vi "Dialog - Select Channel Dialog.vi"(8 "error in (no error)":errorcluster, 9 "Allow Section Selection (F)":bool, 10 "Initial Selection":T1[](array[typedef]) format="%.0x", 11 "Root Item Ref":T1 format="%.0x") -> (0 "error out":errorcluster, 1 "Canceled":bool, 3 "Selected Channel Refs":T1[](array[typedef]) format="%.0x")   [LabVIEW 2016, in "UDP-Custom-Device System Explorer.lvlib"]
doc: "Standard Channel Select Dialog that allows the user to select which TimeStamp channel to use for the header information."
uses:
  UDP-Custom-Device System Explorer.lvlib
  <vilib>/NI Veristand/Custom Device API/Custom Device Item Ref.ctl
  <vilib>/NI VeriStand/Custom Device API/Custom Device API.lvlib
  <vilib>/NI VeriStand/Custom Device Tools/Custom Device Utility Library/Custom Device Utility Library.lvlib
panel:
  in  "Channels":string[](tree)
  in  "Cancel":bool
  in  "OK":bool
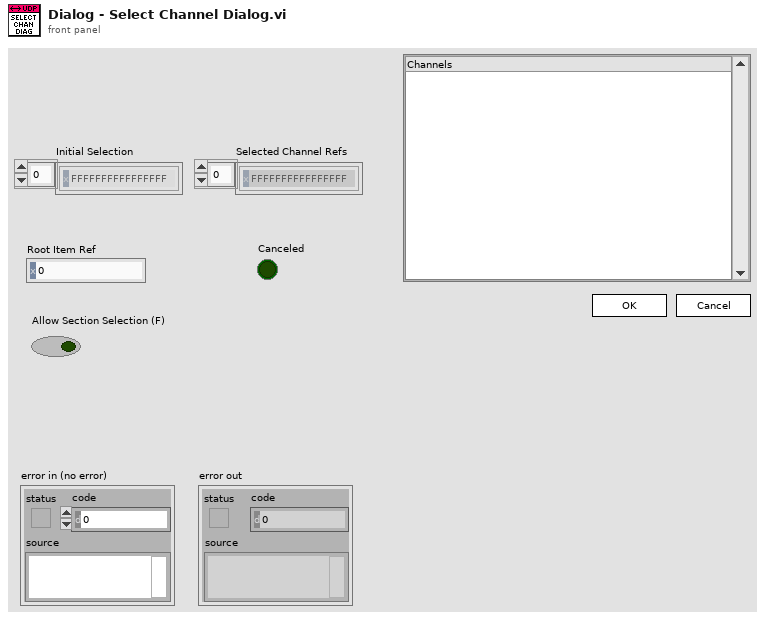
[diagram p1: front panel]
types:
  T1 = typedef "Custom Device API.lvlib/Custom Device Item Ref.ctl" = u64
  T2 = typedef "Custom Device API.lvlib/Custom Device Item Info.ctl" = cluster{"Name":string, "Is Channel":bool, "GUID":string, "Is Waveform":bool}
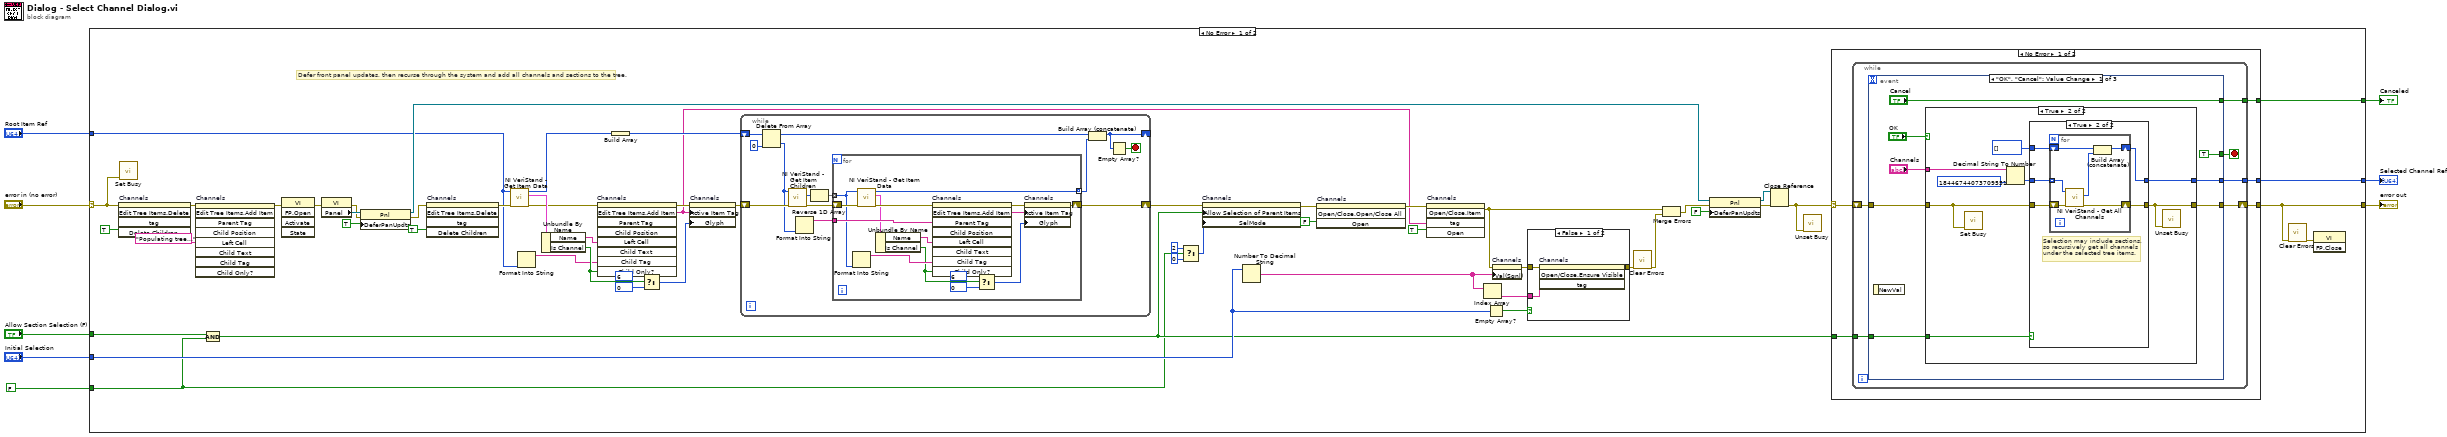
[diagram p0: block diagram]
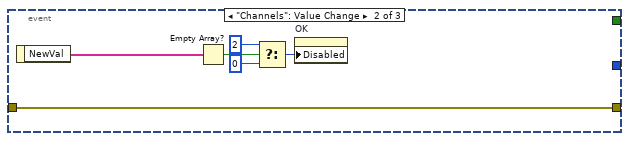
[diagram p5: hidden frame]
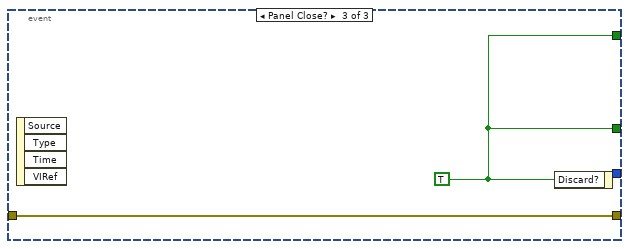
[diagram p6: hidden frame]
diagram:
  n1 = case shown="No Error" "error in (no error)" {
    selector: "error in (no error)" -> [w10 w146]
    tunnel: "Initial Selection" -> [w26 _]
    tunnel: "Allow Section Selection (F)" -> [w16 _]
    tunnel: [w46 w146] -> w5
    tunnel: [w47 _] -> w4
    tunnel: [w44 _] -> w3
    tunnel: "Root Item Ref" -> [w31 _]
    tunnel: FALSE ("Allow Multiple Selection (F)") -> [w11 _]
    frame No Error {
      # "Defer front panel updates, then recurse through the system and add all channels and sections to the tree."
      n2 = invoke on="Channels" class="Tree (strict)" method="Edit Tree Items.Delete"(error in=w10, "Delete Children"=TRUE ("Delete Children?")) -> (error out=w63:errorcluster)  [unwired: 3 in, 4 out]
      n3 = call <vilib>:"Set Busy.vi"("error in (no error)"=w10) -> ()  [unwired: 3 in, 8 out]
      n4 = invoke on="Channels" class="Tree (strict)" method="Edit Tree Items.Add Item"(error in=w63, "Left Cell"="Populating tree..." ("Tag")) -> (error out=w60:errorcluster)  [unwired: 7 in, 8 out]
      n5 = Compound Arithmetic op=AND(w16, w11) -> (w12:bool)
      n6 = invoke class="VI" method="FP.Open"(error in=w60) -> (error out=w58:errorcluster)  [unwired: 4 in, 4 out]
      n7 = property class="VI"(error in=w58) -> (error out=w56:errorcluster, "Panel"=w57:refnum<vi>)  [unwired: 1 in, 1 out]
      n8 = property class="Pnl"(reference=w57, error in=w56, "DeferPanUpdts"=TRUE ("Defer Panel Updates")) -> (reference out=w50:refnum<vi>, error out=w54:errorcluster)
      n9 = invoke on="Channels" class="Tree (strict)" method="Edit Tree Items.Delete"(error in=w54, "Delete Children"=TRUE ("Delete Children?")) -> (error out=w32:errorcluster)  [unwired: 3 in, 4 out]
      n10 = call <vilib>:"NI VeriStand - Get Item Data.vi"("error in (no error)"=w32, "Item Ref in"=w31) -> ("error out"=w35:errorcluster, "Item Info"=w37:T2, "Item Ref out"=w33:T1)  [unwired: 7 out]
      n11 = Format Into String(w31) -> (resulting string=w36:string)  [unwired: 3 in, 1 out]
      n12 = Unbundle By Name(w37) -> ("Name"=w38:string, "Is Channel"=w42:bool)
      n13 = invoke on="Channels" class="Tree (strict)" method="Edit Tree Items.Add Item"(error in=w35, "Left Cell"=w38, "Child Tag"=w36, "Child Only?"=w42) -> (error out=w39:errorcluster, "Edit Tree Items:Add Item"=w17:string)  [unwired: 5 in, 7 out]
      n14 = Build Array(w33) -> (w53:T1[])
      n15 = Select(t=6, s=w42, f=0) -> (s? t:f=w43:i32)
      n16 = property on="Channels" class="Tree (strict)"(error in=w39, "Active Item Tag"=w17, "Glyph"=w43) -> (error out=w34:errorcluster)  [unwired: 1 in, 1 out]
      n17 = while {
        shift-right: [w122] -> w52
        shift-left: w34 -> [w127]
        shift-right: [w126] -> _
        shift-left: w53 -> [w130]
        stop <- w125 stop-if-true
        n18 = Delete From Array(array=w130, index=0) -> (deleted portion=w121:T1, array with subset deleted=w128:T1[])  [unwired: 1 in]
        n19 = call <vilib>:"NI VeriStand - Get Item Children.vi"("error in (no error)"=w127, "Item Ref in"=w121) -> ("error out"=w124:errorcluster, "Child Refs"=w119:T1[])  [unwired: 8 out]
        n20 = Format Into String(w121) -> (resulting string=w120:string)  [unwired: 3 in, 1 out]
        n21 = Reverse 1D Array(array=w119) -> (reversed array=w118:T1[])
        n22 = for {
          shift-right: [w135] -> w122
          shift-left: w124 -> [w144]
          tunnel: w118 -> [w141] mode=indexing
          tunnel: [w142] -> w123 mode=indexing
          tunnel: w120 -> [w145]
          n23 = Format Into String(w141) -> (resulting string=w140:string)  [unwired: 3 in, 1 out]
          n24 = call <vilib>:"NI VeriStand - Get Item Data.vi"("error in (no error)"=w144, "Item Ref in"=w141) -> ("error out"=w143:errorcluster, "Item Info"=w139:T2, "Item Ref out"=w142:T1)  [unwired: 7 out]
          n25 = Unbundle By Name(w139) -> ("Name"=w138:string, "Is Channel"=w132:bool)
          n26 = invoke on="Channels" class="Tree (strict)" method="Edit Tree Items.Add Item"(error in=w143, "Parent Tag"=w145, "Left Cell"=w138, "Child Tag"=w140, "Child Only?"=w132) -> (error out=w137:errorcluster, "Edit Tree Items:Add Item"=w136:string)  [unwired: 4 in, 7 out]
          n27 = Select(t=6, s=w132, f=0) -> (s? t:f=w131:i32)
          n28 = property on="Channels" class="Tree (strict)"(error in=w137, "Active Item Tag"=w136, "Glyph"=w131) -> (error out=w135:errorcluster)  [unwired: 1 in, 1 out]
        }
        n29 = Build Array (concatenate)(w128, w123) -> (w126:T1[])
        n30 = Empty Array?(array=w126) -> (empty?=w125:bool)
      }
      n31 = Select(t=2 ("Selection Mode"), s=w11, f=0 ("Selection Mode")) -> (s? t:f=w13:i32)
      n32 = property on="Channels" class="Tree (strict)"(error in=w52, "Allow Selection of Parent Items"=w12, "SelMode"=w13) -> (error out=w22:errorcluster)  [unwired: 1 in, 1 out]
      n33 = Number To Decimal String(number=w26) -> (decimal integer string=w24:string[])  [unwired: 1 out]
      n34 = invoke on="Channels" class="Tree (strict)" method="Open/Close.Open/Close All"(error in=w22, "Open"=FALSE ("Open?")) -> (error out=w20:errorcluster)  [unwired: 2 in, 3 out]
      n35 = invoke on="Channels" class="Tree (strict)" method="Open/Close.Item"(error in=w20, "tag"=w17, "Open"=TRUE ("Open?")) -> (error out=w18:errorcluster)  [unwired: 2 in, 4 out]
      n36 = Index Array(array=w24) -> (element=w23:string)  [unwired: 1 in]
      n37 = Empty Array?(array=w26) -> (empty?=w25:bool)
      n38 = property on="Channels" class="Tree (strict)"(error in=w18, "Val(Sgnl)"=w24) -> (error out=w28:errorcluster)  [unwired: 1 in, 1 out]
      n39 = case shown="False" w25 {
        tunnel: w28 -> [w66 w67]
        tunnel: [w65 w67] -> w27
        tunnel: w23 -> [w64 _]
        frame False {
          n40 = invoke on="Channels" class="Tree (strict)" method="Open/Close.Ensure Visible"(error in=w66, "tag"=w64) -> (error out=w65:errorcluster)  [unwired: 2 in, 3 out]
        }
        frame True {
        }
      }
      n41 = call <vilib>:"Clear Errors.vi"("error in (no error)"=w27) -> ("error out"=w30:errorcluster)  [unwired: 1 in, 5 out]
      n42 = Merge Errors(w18, w30) -> (w29:errorcluster)
      n43 = property class="Pnl"(reference=w50, error in=w29, "DeferPanUpdts"=FALSE ("Defer Panel Updates")) -> (reference out=w48:refnum<vi>, error out=w49:errorcluster)
      n44 = Close Reference(reference=w48, error in (no error)=w49) -> (error out=w9:errorcluster)
      n45 = call <vilib>:"Unset Busy.vi"("error in (no error)"=w9) -> ()  [unwired: 1 in, 10 out]
      n46 = case shown="No Error" w9 {
        selector: w9 -> [w72 w117]
        tunnel: [w71 w117] -> w46
        tunnel: [w70 _] -> w47
        tunnel: [w69 _] -> w44
        tunnel: w12 -> [w68 _]
        frame No Error {
          n47 = while {
            shift-right: [w77] -> w71
            shift-left: w72 -> [w78]
            tunnel: [w76] -> w70
            tunnel: [w74] -> w69
            tunnel: w68 -> [w73]
            stop <- w75 stop-if-true
            n48 = event shown="[0] \"OK\", \"Cancel\": Value Change" {
              selector: _ -> [_ _ _]
              dyn-events: _ -> [_ _ _]
              timeout: _ -> [_ _ _]
              tunnel: w78 -> [w82 w114 w116]
              tunnel: [w80 w114 w116] -> w77
              tunnel: ["Cancel" _ w115] -> w76
              tunnel: [TRUE ("Discard?") _ w115] -> w75
              tunnel: [w81 _ _] -> w74
              tunnel: w73 -> [w83 _ _]
              event "OK", "Cancel": Value Change {
                n49 = event-data() -> ()  [unwired: 2 out]
                n50 = case shown="True" "OK" {
                  tunnel: "Channels" -> [_ w95]
                  tunnel: w83 -> [_ w93]
                  tunnel: w82 -> [w87 w88]
                  tunnel: [_ w92] -> w81
                  tunnel: [w87 w89] -> w80
                  frame False {
                  }
                  frame True {
                    n51 = call <vilib>:"Set Busy.vi"("error in (no error)"=w88) -> ()  [unwired: 3 in, 8 out]
                    n52 = Decimal String To Number(string=w95, default (0L)=T1 18446744073709551615 ("Device Item Ref")) -> (number=w91:u64[])  [unwired: 2 out]
                    n53 = case shown="True" w93 {
                      tunnel: w88 -> [w96 w102]
                      tunnel: [w97 w100] -> w92
                      tunnel: w91 -> [w97 w99]
                      tunnel: [w96 w98] -> w89
                      tunnel: T1[] [] ("Channel Refs") -> [_ w101]
                      frame False {
                      }
                      frame True {
                        # "Selection may include sections, so recursively get all channels under the selected tree items."
                        n54 = for {
                          shift-right: [w104] -> w100
                          shift-left: w101 -> [w105]
                          shift-right: [w107] -> w98
                          shift-left: w102 -> [w108]
                          tunnel: w99 -> [w106] mode=indexing
                          n55 = call <vilib>:"NI VeriStand - Get All Channels.vi"("error in"=w108, "Section Ref in"=w106) -> ("error out"=w107:errorcluster, "Channel Refs"=w103:T1[])  [unwired: 8 out]
                          n56 = Build Array (concatenate)(w105, w103) -> (w104:T1[])
                        }
                      }
                    }
                    n57 = call <vilib>:"Unset Busy.vi"("error in (no error)"=w89) -> ()  [unwired: 1 in, 10 out]
                  }
                }
              }
              event "Channels": Value Change {
                n58 = event-data() -> ("NewVal"=w113:string[])  [unwired: 1 out]
                n59 = Empty Array?(array=w113) -> (empty?=w112:bool)
                n60 = Select(t=u8 2, s=w112, f=u8 0) -> (s? t:f=w109:u8)
                n61 = property on="OK" class="Bool"("Disabled"=w109) -> ()  [unwired: 2 in, 2 out]
              }
              event Panel Close? {
                w115 = TRUE ("Discard?")
                n62 = event-data() -> ()  [unwired: 5 out]
                n63 = event-data("Discard?"=w115) -> ()  [unwired: 1 in, 1 out]
              }
            }
          }
        }
        frame Error {
        }
      }
      n64 = call <vilib>:"Clear Errors.vi"("error in (no error)"=w46) -> ("error out"=w45:errorcluster)  [unwired: 1 in, 5 out]
      n65 = invoke class="VI" method="FP.Close"(error in=w45) -> ()  [unwired: 2 in, 3 out]
    }
    frame Error {
    }
  }
  "Canceled" <- w4
  "Selected Channel Refs" <- w3
  "error out" <- w5
